vi "VA -Set velocity.vi"(6 "Action":bool, 8 "error in":errorcluster, 9 "Velocity\nset":dbl format="%.2f", 10 "Axis #":i8=1 min=1 max=6 step=1, 11 "Address / Port":i16=1 min=1 max=31 step=1) -> (0 "error out":errorcluster, 1 "Query the current velocity\nsetting - read":string, 2 "Axis # dup":i8=1 min=1 max=6 step=1, 3 "Address / Port dup":i16=1 min=1 max=31 step=1)   [LabVIEW 2014]
panel:
  # "Read"
  # "Write"
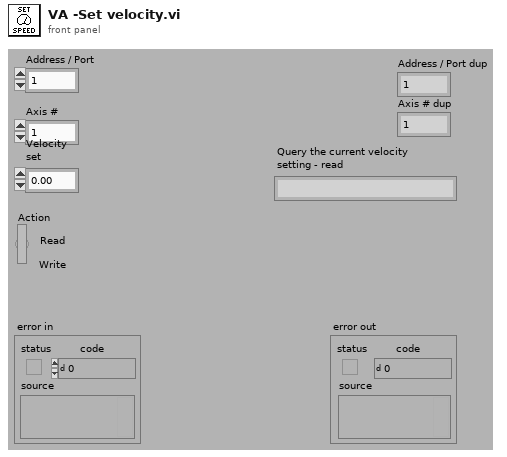
[diagram p1: front panel]
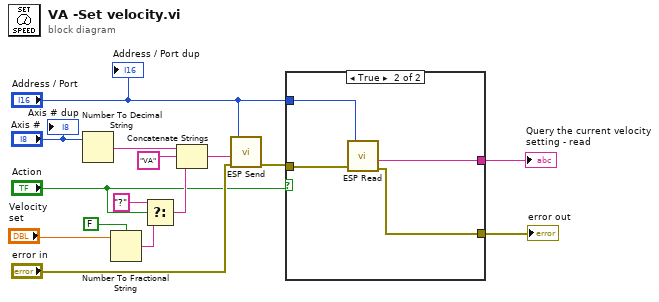
[diagram p0: block diagram]
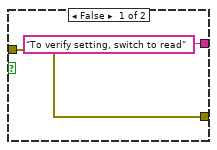
[diagram p2: hidden frame]
diagram:
  n1 = Number To Decimal String(number="Axis #") -> (decimal integer string=w14:string)  [unwired: 1 in]
  n2 = Number To Fractional String(use system decimal point (T)=FALSE, number="Velocity\nset") -> (F-format string=w10:string)  [unwired: 2 in]
  n3 = Select(t="?", s="Action", f=w10) -> (s? t:f=w11:string)
  n4 = Concatenate Strings(w14, "VA" ("Substring"), w11) -> (w12:string)
  n5 = call "ESP Send.vi"("error in"="error in", "Command String"=w12, "Address / Port"="Address / Port") -> ("error out"=w5:errorcluster)  [unwired: 3 in, 1 out]
  n6 = case shown="True" "Action" {
    tunnel: "Address / Port" -> [_ w21]
    tunnel: w5 -> [w17 w20]
    tunnel: [w17 w19] -> w4
    tunnel: ["To verify setting, switch to read" w18] -> w2
    frame False {
    }
    frame True {
      n7 = call "ESP Read.vi"("error in"=w20, "Address / Port"=w21) -> ("error out"=w19:errorcluster, "Response String"=w18:string)  [unwired: 3 in, 1 out]
    }
  }
  "error out" <- w4
  "Query the current velocity\nsetting - read" <- w2
  "Address / Port dup" <- "Address / Port"
  "Axis # dup" <- "Axis #"
